vi "NodosPropiedad19-05-23.vi"() -> ()   [LabVIEW 2020]
panel:
  in  "stop":bool
  out "Temperatura":cluster{dbl, "Limite Superior":dbl}(graph)
  out "String":string
  out "#Muestreo":i32
  out "Fuera de Rango":bool
  in  "Limite de muestreo":i32
  in  "Limite Superior":dbl
  in  "T.Muestreo":dbl
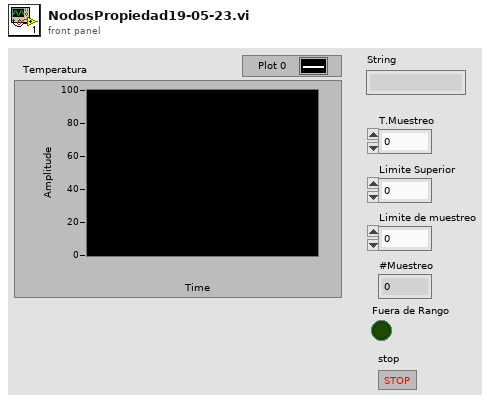
[diagram p1: front panel]
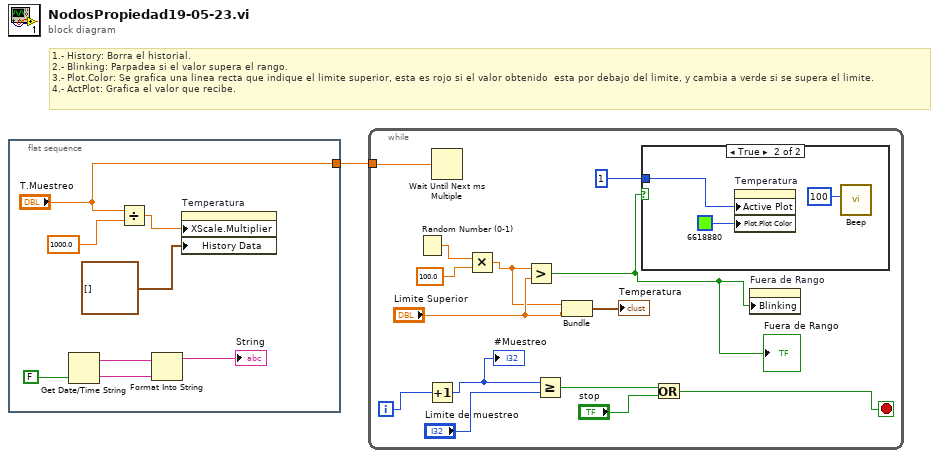
[diagram p0: block diagram]
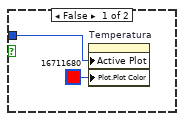
[diagram p2: hidden frame]
diagram:
  # "1.- History: Borra el historial.\n2.- Blinking: Parpadea si el valor supera el rango.\n3.- Plot.Color: Se grafica una linea recta que indique el limite superior, esta es rojo si el valor obtenido  esta por debajo del limite, y cambia a verde si se supera el limite.\n4.- ActPlot: Grafica el valor que recibe."
  n1 = flat-sequence {
    tunnel: ["T.Muestreo"] -> w1
    frame #0 {
      n2 = Get Date/Time String(want seconds? (F)=FALSE) -> (date string=w7:string, time string=w6:string)  [unwired: 2 in]
      n3 = Divide(x="T.Muestreo", y=1000.0) -> (x/y=w8:dbl)
      n4 = Format Into String(initial string=w7, w6) -> (resulting string=→"String":string)  [unwired: 2 in, 1 out]
      n5 = property on="Temperatura" class="WFChart (strict)"("XScale.Multiplier"=w8, "History Data"=cluster{dbl, "Limite Superior":dbl}[] []) -> ()  [unwired: 2 in, 2 out]
    }
  }
  n6 = while {
    tunnel: w1 -> [w23]
    i -> [w17]
    stop <- w15 stop-if-true
    n7 = Random Number (0-1)() -> (number: 0 to 1=w22:dbl)
    n8 = Increment(x=w17) -> (x+1=w14:i32)
    "#Muestreo" <- w14
    n9 = Wait Until Next ms Multiple(millisecond multiple=w23) -> ()  [unwired: 1 out]
    n10 = Multiply(x=w22, y=100.0) -> (x*y=w19:dbl)
    n11 = Greater?(x=w19, y="Limite Superior") -> (0:w11:bool)
    "Fuera de Rango" <- w11
    n12 = Greater Or Equal?(x=w14, y="Limite de muestreo") -> (x >= y?=w16:bool)
    n13 = Bundle(w19, "Limite Superior"="Limite Superior") -> (→"Temperatura":cluster{dbl, "Limite Superior":dbl})  [unwired: 1 in]
    n14 = case shown="True" w11 {
      tunnel: 1 -> [w25 w28]
      frame False {
        n15 = property on="Temperatura" class="WFChart (strict)"("Active Plot"=w25, "Plot.Plot Color"=u32 16711680) -> ()  [unwired: 2 in, 2 out]
      }
      frame True {
        n16 = property on="Temperatura" class="WFChart (strict)"("Active Plot"=w28, "Plot.Plot Color"=u32 6618880) -> ()  [unwired: 2 in, 2 out]
        n17 = call <vilib>:"Beep.vi"("duration (msec)"=u32 100) -> ()  [unwired: 11 in]
      }
    }
    n18 = Or(x=w16, y="stop") -> (x .or. y?=w15:bool)
    n19 = property on="Fuera de Rango" class="Bool (strict)"("Blinking"=w11) -> ()  [unwired: 2 in, 2 out]
  }
